vi "AddonMotors Controller.vi"(8 "error in":errorcluster) -> ()   [LabVIEW 2015]
doc: "This VI executes continuously carrying out the current operation and responding to updates or new operations. It will often contain the timing or control code that is difficult to place directly in TeleOp. This VI generally opens all sensors and motors and isolates the rest of the robot code from knowing how the operations are carried out."
uses:
  AddonMotors Setpoints.ctl
  AddonMotors Operations.ctl
  Framework/Robot Global Data.vi
panel:
  out "Clock":u32(knob) scale=0.0..10000.0
  out "Current\nCmd":string
  # "Tip: It may be helpful to observe inputs and sensor values.\nYou may also want to display tuning or debugging controls."
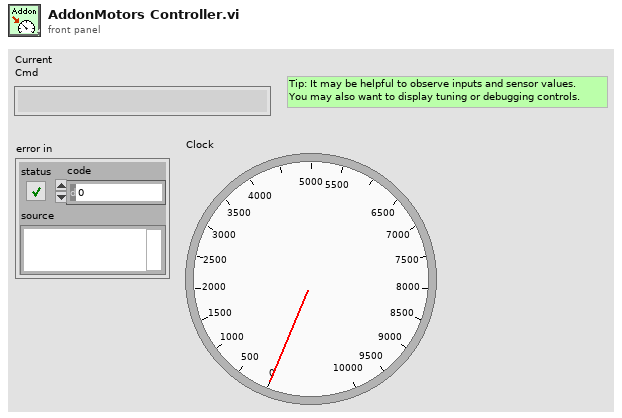
[diagram p1: front panel]
types:
  T1 = typedef "AddonMotors Setpoints.ctl" = cluster{"Operation":T2, "Setpoint":dbl, "Duration":dbl, "Motor ID":dbl}
  T2 = typedef "AddonMotors Operations.ctl" = enum16{"Reserve", "Read Current", "Immediate", "Angle (Position)", "Speed", "Angle Increments (Position)"}
  T3 = typedef "Command Status Info.ctl" = cluster{"Name":string, "Status":T4, "notifier out":T5}
  T4 = typedef "Completion Status.ctl" = enum16{"Successful", "Aborted", "Incomplete"}
  T5 = typedef "Completion Notifier.ctl" = refnum<notifier>
  T6 = cluster{"Default Command":T1, "Command Timing":cluster{"Start Time (ms)":u32, "Iterations":i32}, "Command Arguments":cluster{"Command Info":T3, "Description":string, "Default Command":T1, "notifier out":refnum<notifier>, "Subsystem Name":string}}
  T7 = typedef "Motor Ref Array Type Def.ctl" = T8[]
  T8 = typedef "Detailed Motor Type Def.ctl" = cluster{"MotorRef":T9, "Encoder Ticks Per Rev":dbl, "Set Position":dbl}
  T9 = typedef "WPI_MotorControlDeviceRef.ctl" = cluster{"DeviceStatus":errorcluster, "Type":T10, "PWM":cluster{"PWM Channel":T11, "DeadBand":T12}, "CAN":cluster{"Device Number":u8, "Control Mode":T13, "Semaphore":T14, "Max Vout":dbl, "TalonSRX Control Mode":T15}, "Invert":bool}
  T10 = typedef "WPI_MotorControlType.ctl" = enum16{"PWM", "CAN", "CANTalonSRX"}
  T11 = typedef "FPGA_DIOPWMChannel.ctl" = enum8{"PWM 0", "PWM 1", "PWM 2", "PWM 3", "PWM 4", "PWM 5", "PWM 6", "PWM 7", "PWM 8", "PWM 9", "PWM MXP 0", "PWM MXP 1", "PWM MXP 2", "PWM MXP 3", "PWM MXP 4", "PWM MXP 5", "PWM MXP 6", "PWM MXP 7", "PWM MXP 8", "PWM MXP 9", "Invalid"}
  T12 = typedef "WPI_PWMDeadband.ctl" = cluster{"Name":string, "maxPositivePwm":i32, "minPositivePwm":i32, "centerPwm":i32, "maxNegativePwm":i32, "minNegativePwm":i32, "angularRange":u16}
  T13 = typedef "WPI_CANJaguar_ControlMode.ctl" = enum8{"Percent VBus", "Current", "Speed", "Position", "Voltage"}
  T14 = typedef "Semaphore RefNum" = refnum<k1>
  T15 = typedef "WPI_CANTalonSRX_APIControlMode.ctl" = enum8{"Percent VBus", "Speed", "Position", "Slave", "Unchanged / Invalid", "Voltage Compensation", "Current", "Motion Profile"}
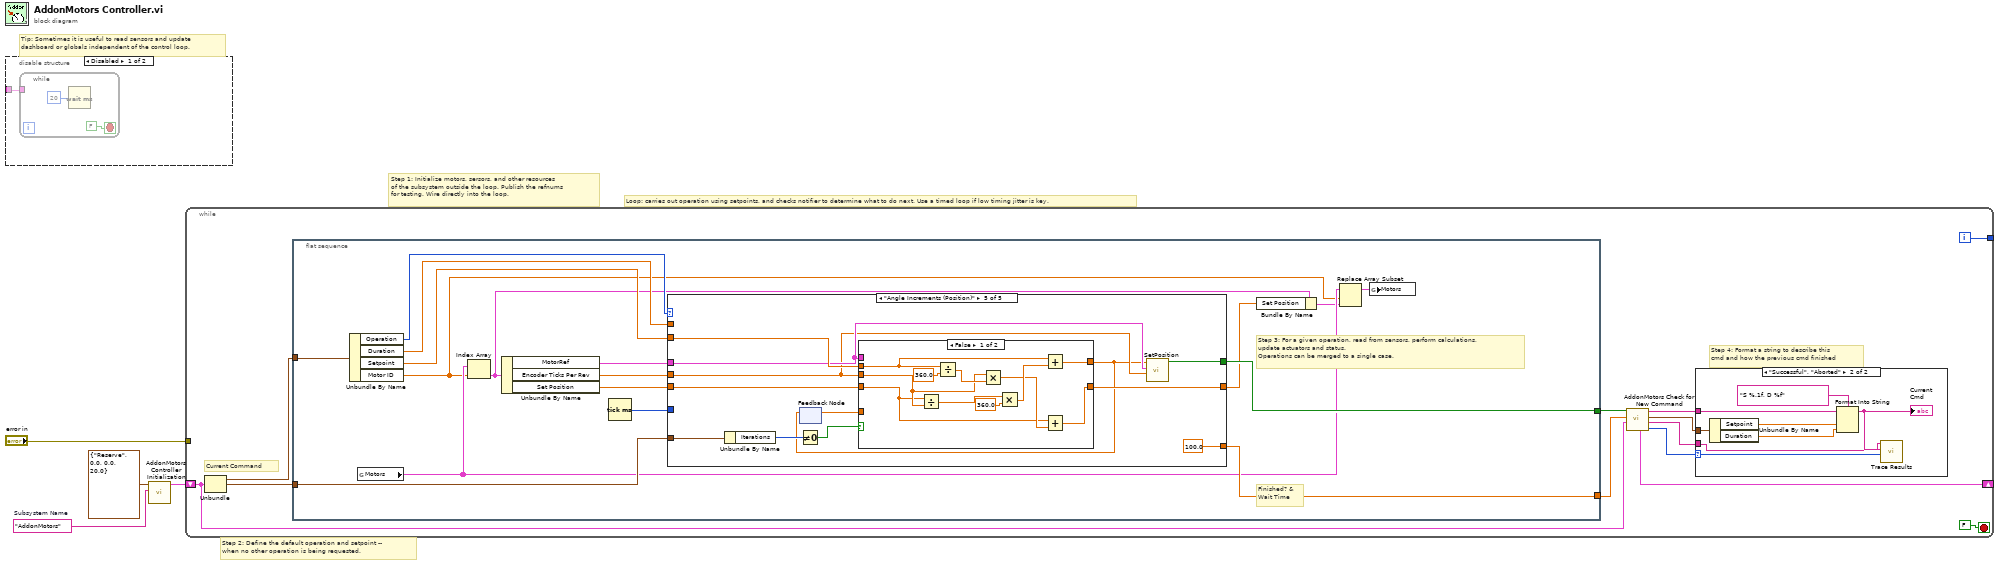
[diagram p0: block diagram]
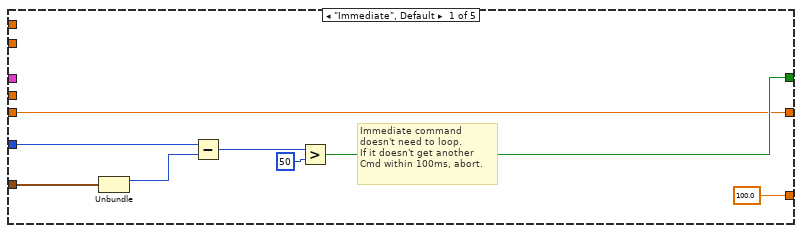
[diagram p3: hidden frame]
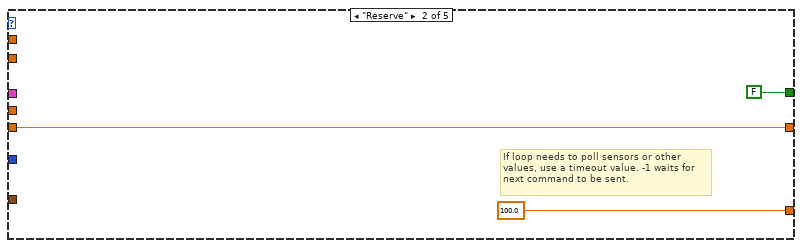
[diagram p4: hidden frame]
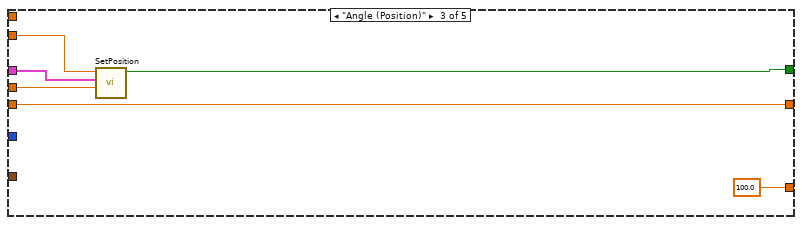
[diagram p5: hidden frame]
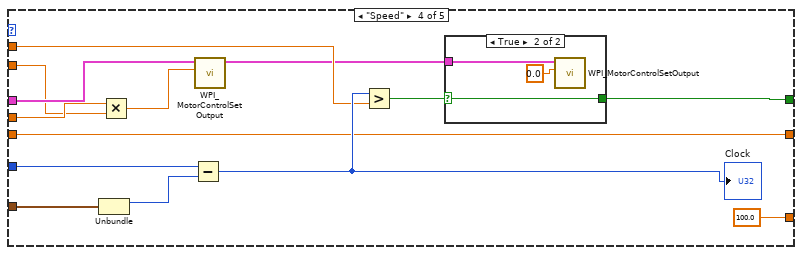
[diagram p6: hidden frame]
diagram:
  w2 = "AddonMotors"  # Subsystem Name
  # "Tip: Sometimes it is useful to read sensors and update\ndashboard or globals independent of the control loop."
  # "Step 2: Define the default operation and setpoint --\nwhen no other operation is being requested."
  # "Step 1: Initialize motors, sersors, and other resources\nof the subsystem outside the loop. Publish the refnums\nfor testing. Wire directly into the loop."
  # "Loop: carries out operation using setpoints, and checks notifier to determine what to do next. Use a timed loop if low timing jitter is key."
  n1 = disable-structure shown="Disabled" {
    disable-tunnel: _ -> [w5 _]
    frame Disabled {
      n2 = while {
        tunnel: w5 -> [_]
        stop <- FALSE stop-if-true
        n3 = Wait (ms)(milliseconds to wait=u32 20) -> ()  [unwired: 1 out]
      }
    }
    frame Enabled {
    }
  }
  n4 = call "AddonMotors Controller Initialization.vi"("Subsystem Name"=w2, "Default Command"=T1 {"Operation"=enum."Reserve", "Setpoint"=0.0, "Duration"=0.0, "Motor ID"=20.0}) -> ("Command Info"=w3:T6)  [unwired: 9 in]
  n5 = while {
    shift-right: [w14] -> _
    shift-left: w3 -> [w15]
    tunnel: [w18] -> _
    tunnel: "error in" -> [_]
    i -> [w18]
    stop <- FALSE stop-if-true
    # "Step 4: Format a string to describe this\ncmd and how the previous cmd finished"
    # "Current Command"
    n6 = Unbundle(w15) -> ("Default Command"=w17:T1, "Command Timing"=w16:cluster{"Start Time (ms)":u32, "Iterations":i32})  [unwired: 1 out]
    n7 = flat-sequence {
      tunnel: w17 -> [w36]
      tunnel: w16 -> [w32]
      tunnel: [w30] -> w13
      tunnel: [w29] -> w12
      frame #0 {
        # "Finished? &\nWait Time"
        # "Step 3: For a given operation, read from sensors, perform calculations,\nupdate actuators and status.\nOperations can be merged to a single case."
        n8 = Unbundle By Name(w36) -> ("Operation"=w35:T2, "Duration"=w34:dbl, "Setpoint"=w31:dbl, "Motor ID"=w21:dbl)
        n9 = global read "Robot Global Data.vi" "Motors"() -> (w23:T7)
        n10 = Index Array(array=w23, index=w21) -> (element=w25:T8)
        n11 = Unbundle By Name(w25) -> ("MotorRef"=w28:T9, "Encoder Ticks Per Rev"=w27:dbl, "Set Position"=w26:dbl)
        n12 = Tick Count (ms)() -> (millisecond timer value=w33:u32)
        n13 = case shown="\"Angle Increments (Position)\"" w35 {
          tunnel: [100.0 100.0 100.0 100.0 100.0] -> w29
          tunnel: [w38 FALSE ("ignore previous (F)") w51 w56 w73] -> w30
          tunnel: w32 -> [w40 _ _ w60 w80]
          tunnel: w34 -> [_ _ _ w58 _]
          tunnel: w33 -> [w39 _ _ w61 _]
          tunnel: w31 -> [_ _ w53 w64 w82]
          tunnel: w28 -> [_ _ w52 w67 w76]
          tunnel: w27 -> [_ _ w49 w65 w75]
          tunnel: w26 -> [w37 w45 w48 w54 w78]
          tunnel: [w37 w45 w48 w54 w77] -> w24
          frame "Immediate", Default {
            # "Immediate command\ndoesn't need to loop.\nIf it doesn't get another\nCmd within 100ms, abort."
            n14 = Unbundle(w40) -> ("Start Time (ms)"=w43:u32)  [unwired: 1 out]
            n15 = Subtract(x=w39, y=w43) -> (x-y=w42:u32)
            n16 = Greater?(x=w42, y=u8 50 ("Left Motor")) -> (0:w38:bool)
          }
          frame "Reserve" {
            # "If loop needs to poll sensors or other\nvalues, use a timeout value. -1 waits for\nnext command to be sent."
          }
          frame "Angle (Position)" {
            n17 = call "SetPosition.vi"("Encoder Ticks Per Rev"=w49, "MotorRef"=w52, "Setpoint"=w53) -> ("Done?"=w51:bool)  [unwired: 8 in]
          }
          frame "Speed" {
            n18 = Unbundle(w60) -> ("Start Time (ms)"=w63:u32)  [unwired: 1 out]
            n19 = Multiply(x=w65, y=w64) -> (x*y=w66:dbl)
            n20 = Subtract(x=w61, y=w63) -> (x-y=w62:u32)
            "Clock" <- w62
            n21 = call <vilib>:"WPI_MotorControlSetOutput.vi"("Output"=w66, "MotorControlDevRef"=w67) -> ("MotorControlDevRef"=w55:T9)  [unwired: 7 in, 2 out]
            n22 = Greater?(x=w62, y=w58) -> (0:w57:bool)
            n23 = case shown="True" w57 {
              selector: w57 -> [w68 w71]
              tunnel: [w68 w71] -> w56
              tunnel: w55 -> [_ w70]
              frame False {
              }
              frame True {
                n24 = call <vilib>:"WPI_MotorControlSetOutput.vi"("Output"=0.0, "MotorControlDevRef"=w70) -> ()  [unwired: 7 in, 3 out]
              }
            }
          }
          frame "Angle Increments (Position)" {
            n25 = Unbundle By Name(w80) -> ("Iterations"=w79:i32)
            n26 = Not Equal To 0?(x=w79) -> (x != 0?=w81:bool)
            n27 = feedback #1() -> (w74:dbl)  [unwired: 1 in]
            n28 = case shown="False" w81 {
              tunnel: [w94 w95] -> w72
              tunnel: w75 -> [w88 _]
              tunnel: w76 -> [_ _]
              tunnel: w82 -> [w87 _]
              tunnel: w74 -> [_ w95]
              tunnel: w78 -> [w84 w96]
              tunnel: [w85 w96] -> w77
              frame False {
                n29 = Divide(x=w84, y=w88) -> (x/y=w93:dbl)
                n30 = Divide(x=w87, y=360.0) -> (x/y=w89:dbl)
                n31 = Multiply(x=w88, y=w89) -> (x*y=w86:dbl)
                n32 = Multiply(x=w93, y=360.0) -> (x*y=w91:dbl)
                n33 = Add(x=w87, y=w91) -> (x+y=w94:dbl)
                n34 = Add(x=w84, y=w86) -> (x+y=w85:dbl)
              }
              frame True {
              }
            }
            n35 = feedback-in #1(w72) -> ()
            n36 = call "SetPosition.vi"("Encoder Ticks Per Rev"=w75, "MotorRef"=w76, "Setpoint"=w72) -> ("Done?"=w73:bool)  [unwired: 8 in]
          }
        }
        n37 = Bundle By Name(cluster=w25, "Set Position"=w24) -> (w22:T8)
        n38 = Replace Array Subset(array=w23, new element=w22, index=w21) -> (w20:T7)
        n39 = global write "Robot Global Data.vi" "Motors"(w20) -> ()
      }
    }
    n40 = call "AddonMotors Check for New Command.vi"("Current Command"=w15, "Wait time (ms)"=w12, "Finished?"=w13) -> ("Completion"=w8:T4, "Subsystem Name"=w9:string, "Current Command"=w10:T1, "Initial Trace String"=w11:string, "NextCommand"=w14:T6)  [unwired: 4 in]
    n41 = case shown="\"Successful\", \"Aborted\"" w8 {
      selector: w8 -> [_ w104]
      tunnel: w11 -> [_ w100]
      tunnel: w10 -> [_ w101]
      tunnel: w9 -> [_ w97]
      frame "Incomplete", Default {
        # "Continuing current command"
      }
      frame "Successful", "Aborted" {
        # "Report and setup for next command"
        n42 = Unbundle By Name(w101) -> ("Setpoint"=w103:dbl, "Duration"=w98:dbl)
        n43 = Format Into String(format string="S %.1f, D %f", initial string=w100, w103, w98) -> (resulting string=w99:string)  [unwired: 1 in, 1 out]
        "Current\nCmd" <- w99
        n44 = call <vilib>:"Trace Results.vi"("Status of previous command"=w104, "Description"=w99, "Subsystem"=w97) -> ()  [unwired: 9 in]
      }
    }
  }
